vi "configure.vi"(8 "error in (no error)":errorcluster, 11 "GenericPlugin in":refnum<class "SignalWriterMH110203USBStepperMotor.lvclass">) -> (0 "error out":errorcluster, 3 "GenericPlugin out":refnum<class "SignalWriterMH110203USBStepperMotor.lvclass">)   [LabVIEW 2010, in "SignalWriterMH110203USBStepperMotor.lvclass"]
doc: "The dynamic dispatch version of this VI loads and displays the configuration file associated with the plug-in object. The user modify and save the configuration data."
uses:
  SignalWriterMH110203USBStepperMotor.lvclass
  common/classes/ErrorController/ErrorController/class_data.vi
  common/classes/GenericComponent/GenericComponent/GenericComponent.lvclass
  common/classes/ErrorController/ErrorController/ErrorController.lvclass
panel:
  in  "maximum output value":dbl=1.0 caption="to"
  in  "minimum output value":dbl=-1.0 caption="from"
  in  "axis":i32(ring) items=["x-axis", "y-axis"]
  in  "step":u8(slide) scale=0.0..3.0
  in  "speed":dbl(slide)=677.1428571428571 min=3.815628815628816 max=1250.0 scale=15.262515262515263..5000.0
  in  "cancel button":bool
  in  "save button":bool
  out "configuration":string
  # "Configure MH101129USBStepperMotor"
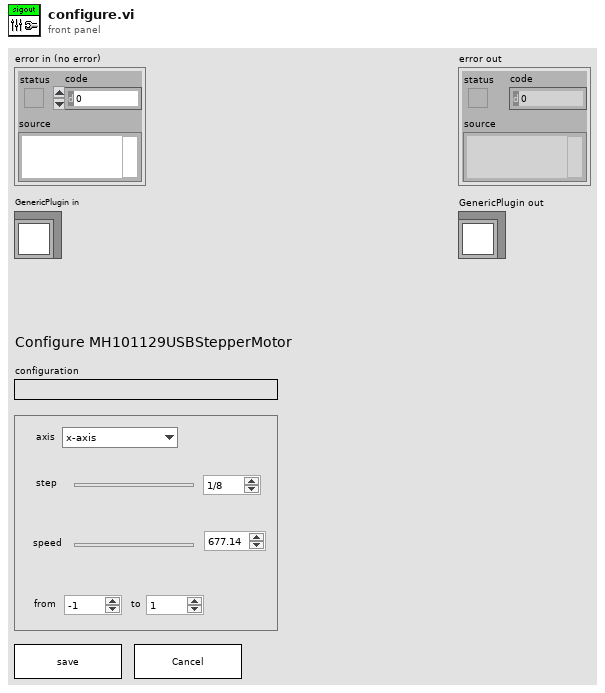
[diagram p1: front panel]
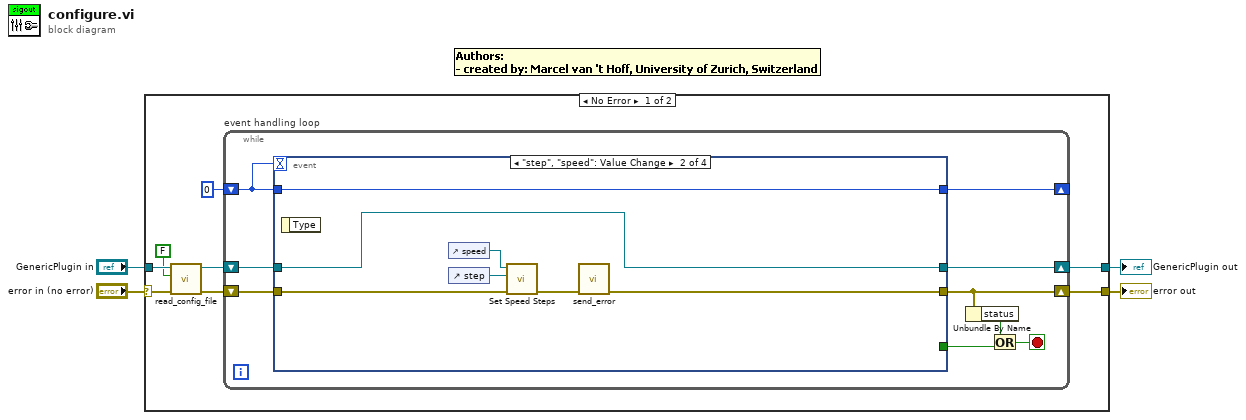
[diagram p0: block diagram]
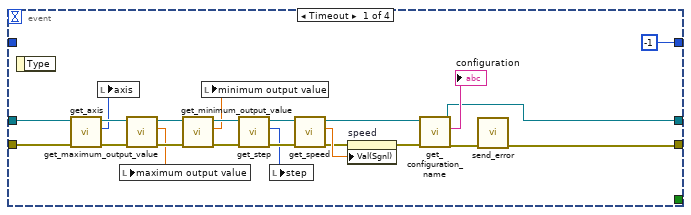
[diagram p2: hidden frame]
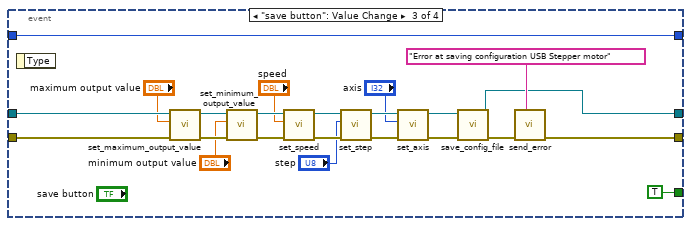
[diagram p3: hidden frame]
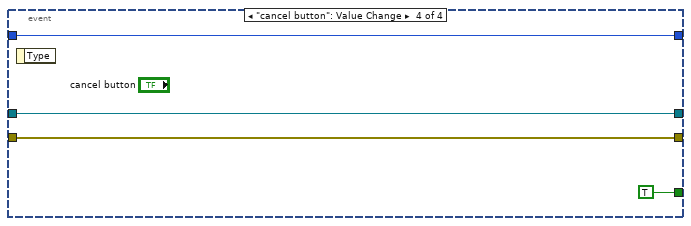
[diagram p4: hidden frame]
diagram:
  n1 = case shown="No Error" "error in (no error)" {
    selector: "error in (no error)" -> [w11 w79]
    tunnel: [w5 w79] -> w3
    tunnel: "GenericPlugin in" -> [w10 w80]
    tunnel: [w6 w80] -> w1
    frame No Error {
      n2 = call-dynamic "read_config_file.vi"("error in (no error)"=w11, "force load?"=FALSE, "GenericPlugin in"=w10) -> ("error out"=w7:errorcluster, "GenericPlugin out"=w8:refnum<class "SignalWriterMH110203USBStepperMotor.lvclass">)  [unwired: 7 out]
      n3 = while "event handling loop" {
        shift-right: [w21] -> _
        shift-left: 0 -> [w20]
        shift-right: [w16] -> w5
        shift-left: w7 -> [w18]
        shift-right: [w17] -> w6
        shift-left: w8 -> [w19]
        stop <- w13 stop-if-true
        n4 = event shown="[1] \"step\", \"speed\": Value Change" {
          selector: _ -> [_ _ _ _]
          dyn-events: _ -> [_ _ _ _]
          timeout: w20 -> [_ _ _ _]
          tunnel: [-1 w51 w74 w78] -> w21
          tunnel: w20 -> [_ w51 w74 w78]
          tunnel: w19 -> [w43 w50 w73 w77]
          tunnel: w18 -> [w40 w48 w68 w76]
          tunnel: [w23 w50 w60 w77] -> w17
          tunnel: [w22 w49 w58 w76] -> w16
          tunnel: [_ _ TRUE TRUE] -> w14
          event Timeout {
            n5 = event-data() -> ()  [unwired: 1 in, 1 out]
            n6 = call-dynamic "get_axis.vi"("error in (no error)"=w40, "SignalWriterMH110203USBStepperMotor in"=w43) -> ("error out"=w39:errorcluster, "axis"=w28:i32, "SignalWriterMH110203USBStepperMotor out"=w42:refnum<class "SignalWriterMH110203USBStepperMotor.lvclass">)  [unwired: 7 in]
            n7 = local write "axis"(w28) -> ()
            n8 = call-dynamic "get_maximum_output_value.vi"("error in (no error)"=w39, "GenericWriteSignals.lvclass in"=w42) -> ("error out"=w38:errorcluster, "maximum output value"=w27:dbl, "GenericWriteSignals.lvclass out"=w41:refnum<class "SignalWriterMH110203USBStepperMotor.lvclass">)  [unwired: 7 in]
            n9 = local write "maximum output value"(w27) -> ()
            n10 = call-dynamic "get_minimum_output_value.vi"("error in (no error)"=w38, "GenericWriteSignals.lvclass in"=w41) -> ("error out"=w35:errorcluster, "minimum output value"=w26:dbl, "GenericWriteSignals.lvclass out"=w36:refnum<class "SignalWriterMH110203USBStepperMotor.lvclass">)  [unwired: 7 in]
            n11 = local write "minimum output value"(w26) -> ()
            n12 = call-dynamic "get_step.vi"("error in (no error)"=w35, "SignalWriterMH110203USBStepperMotor in"=w36) -> ("error out"=w34:errorcluster, "step"=w25:u8, "SignalWriterMH110203USBStepperMotor out"=w33:refnum<class "SignalWriterMH110203USBStepperMotor.lvclass">)  [unwired: 7 in]
            n13 = local write "step"(w25) -> ()
            n14 = call-dynamic "get_speed.vi"("error in (no error)"=w34, "SignalWriterMH110203USBStepperMotor in"=w33) -> ("error out"=w30:errorcluster, "speed"=w31:dbl, "SignalWriterMH110203USBStepperMotor out"=w32:refnum<class "SignalWriterMH110203USBStepperMotor.lvclass">)  [unwired: 7 in]
            n15 = property on="speed" class="Slide (strict)"(error in=w30, "Val(Sgnl)"=w31) -> (error out=w29:errorcluster)  [unwired: 1 in, 1 out]
            n16 = call "get_configuration_name.vi"("error in (no error)"=w29, "GenericPlugin.lvclass in"=w32) -> ("error out"=w24:errorcluster, "configuration name"=→"configuration":string, "GenericPlugin.lvclass out"=w23:refnum<class "SignalWriterMH110203USBStepperMotor.lvclass">)  [unwired: 7 in]
            n17 = call "send_error.vi"("error in (no error)"=w24) -> ("error out"=w22:errorcluster)  [unwired: 10 in]
          }
          event "step", "speed": Value Change {
            n18 = event-data() -> ()  [unwired: 1 in, 1 out]
            n19 = control-ref of="speed"() -> (w46:refnum<vi>)
            n20 = control-ref of="step"() -> (w45:refnum<vi>)
            n21 = call "Set Speed Steps.vi"("error in (no error)"=w48, "Step ref in"=w45, "Speed ref in"=w46) -> ("error out"=w47:errorcluster)  [unwired: 8 in]
            n22 = call "send_error.vi"("error in (no error)"=w47) -> ("error out"=w49:errorcluster)  [unwired: 10 in]
          }
          event "save button": Value Change {
            n23 = event-data() -> ()  [unwired: 1 in, 1 out]
            n24 = call-dynamic "set_maximum_output_value.vi"("error in (no error)"=w68, "maximum output value"="maximum output value", "GenericWriteSignals.lvclass in"=w73) -> ("error out"=w67:errorcluster, "GenericWriteSignals.lvclass out"=w72:refnum<class "SignalWriterMH110203USBStepperMotor.lvclass">)  [unwired: 7 in]
            n25 = call-dynamic "set_minimum_output_value.vi"("error in (no error)"=w67, "minimum output value"="minimum output value", "GenericWriteSignals.lvclass in"=w72) -> ("error out"=w66:errorcluster, "GenericWriteSignals.lvclass out"=w71:refnum<class "SignalWriterMH110203USBStepperMotor.lvclass">)  [unwired: 7 in]
            n26 = call-dynamic "set_speed.vi"("error in (no error)"=w66, "speed"="speed", "SignalWriterMH110203USBStepperMotor in"=w71) -> ("error out"=w65:errorcluster, "SignalWriterMH110203USBStepperMotor out"=w70:refnum<class "SignalWriterMH110203USBStepperMotor.lvclass">)  [unwired: 7 in]
            n27 = call-dynamic "set_step.vi"("error in (no error)"=w65, "step"="step", "SignalWriterMH110203USBStepperMotor in"=w70) -> ("error out"=w64:errorcluster, "SignalWriterMH110203USBStepperMotor out"=w69:refnum<class "SignalWriterMH110203USBStepperMotor.lvclass">)  [unwired: 7 in]
            n28 = call-dynamic "set_axis.vi"("error in (no error)"=w64, "axis"="axis", "SignalWriterMH110203USBStepperMotor in"=w69) -> ("error out"=w63:errorcluster, "SignalWriterMH110203USBStepperMotor out"=w62:refnum<class "SignalWriterMH110203USBStepperMotor.lvclass">)  [unwired: 7 in]
            n29 = call-dynamic "save_config_file.vi"("error in (no error)"=w63, "GenericPlugin in"=w62) -> ("error out"=w59:errorcluster, "GenericPlugin out"=w60:refnum<class "SignalWriterMH110203USBStepperMotor.lvclass">)  [unwired: 2 in, 6 out]
            n30 = call "send_error.vi"("additional message"="Error at saving configuration USB Stepper motor", "error in (no error)"=w59) -> ("error out"=w58:errorcluster)  [unwired: 9 in]
          }
          event "cancel button": Value Change {
            n31 = event-data() -> ()  [unwired: 1 in, 1 out]
          }
        }
        n32 = Unbundle By Name(w16) -> ("status"=w15:bool)
        n33 = Or(x=w15, y=w14) -> (x .or. y?=w13:bool)
      }
    }
    frame Error {
    }
  }
  "error out" <- w3
  "GenericPlugin out" <- w1
